vi "Read Offset Angle.vi"(8 "error in (no error)":errorcluster, 11 "servo motor in":refnum<class "NI_Robotics_Starter Kit Servo Motor.lvclass">) -> (0 "error out":errorcluster, 2 "ccw offset angle (rad)":dbl, 3 "servo motor out":refnum<class "NI_Robotics_Starter Kit Servo Motor.lvclass">)   [LabVIEW 2017, in "NI_Robotics_Starter Kit Servo Motor.lvclass"]
uses:
  <vilib>/robotics/Starter Kit/Servo Motor/NI_Robotics_Starter Kit Servo Motor.lvclass
  <vilib>/robotics/Starter Kit/Servo Motor/NI_Robotics_Starter Kit Servo Motor.lvclass/NI_Robotics_Starter Kit Servo Motor.ctl
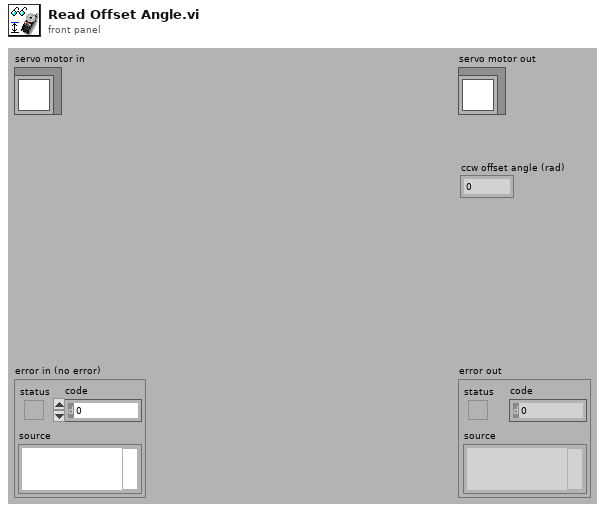
[diagram p1: front panel]
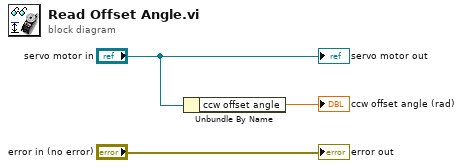
[diagram p0: block diagram]
diagram:
  n1 = Unbundle By Name("servo motor in") -> ("ccw offset angle"=→"ccw offset angle (rad)":dbl)
  "error out" <- "error in (no error)"
  "servo motor out" <- "servo motor in"
